vi "System Semaphore Query.vi"(0 "SemaphoreHandle":u16 format="%.0x", 1 "error in (no error)":errorcluster) -> (2 "State String":string, 3 "State":i32, 4 "PreviousCount":i32, 5 "error out":errorcluster)   [LabVIEW 2011]
uses:
  kernel32.dll
panel:
  in  "PreviousCount in":i32
  # "Returns 0, 1, or -1 for Semaphore Unlocked, Locked, or Non-existent"
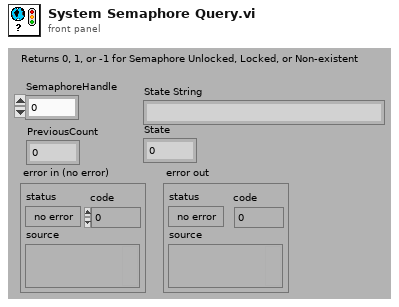
[diagram p1: front panel]
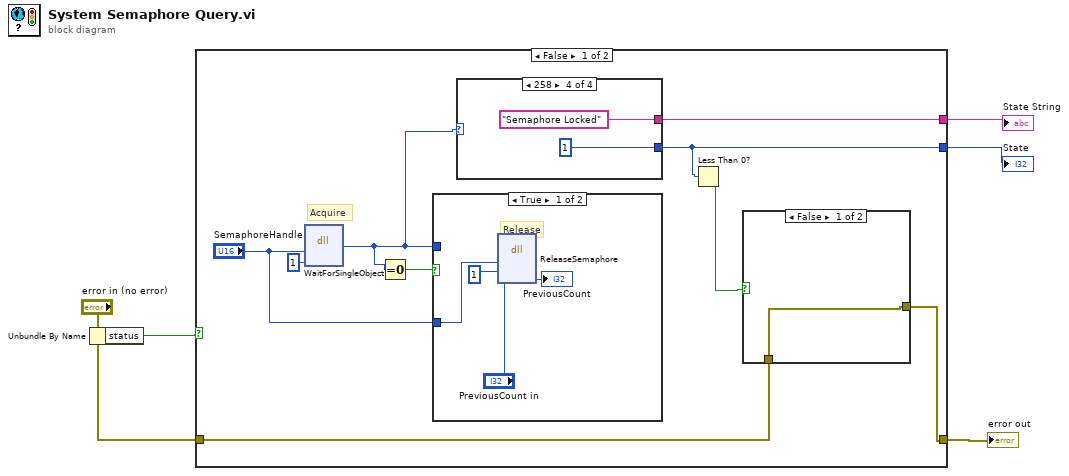
[diagram p0: block diagram]
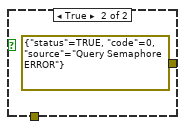
[diagram p3: hidden frame]
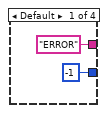
[diagram p4: hidden frame]
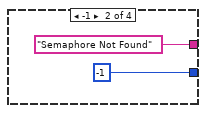
[diagram p5: hidden frame]
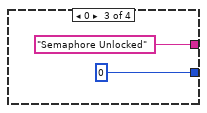
[diagram p6: hidden frame]
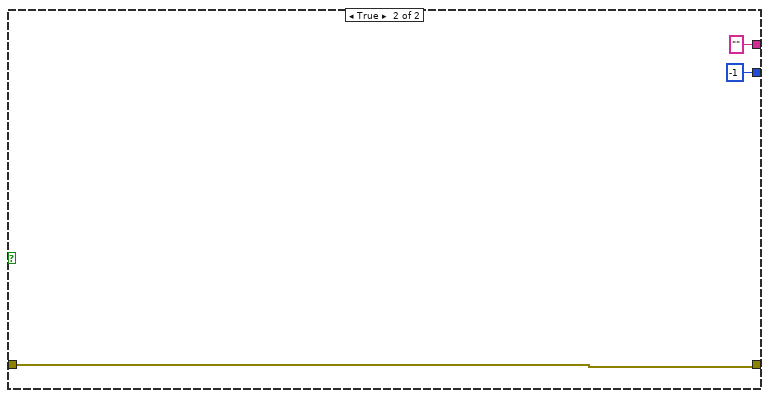
[diagram p7: hidden frame]
diagram:
  n1 = Unbundle By Name("error in (no error)") -> ("status"=w4:bool)
  n2 = case shown="False" w4 {
    tunnel: "error in (no error)" -> [w9 w31]
    tunnel: [w8 w31] -> w1
    tunnel: [w12 ""] -> w3
    tunnel: [w11 -1] -> w2
    frame False {
      # "Acquire"
      n3 = dll-call lib="kernel32.dll" fn="WaitForSingleObject"("SemaphoreHandle"="SemaphoreHandle", "Timeoutms"=u16 1) -> (w7:i16)  [unwired: 5 in, 2 out]
      n4 = Equal To 0?(x=w7) -> (x = 0?=w6:bool)
      n5 = case shown="True" w6 {
        tunnel: "SemaphoreHandle" -> [w18 _]
        tunnel: w7 -> [_ _]
        frame True {
          # "Release"
          n6 = dll-call lib="kernel32.dll" fn="ReleaseSemaphore"("SemaphoreHandle"=w18, "ReleaseCount"=1, "PreviousCount"="PreviousCount in") -> ("PreviousCount"=→"PreviousCount":i32)  [unwired: 6 in, 2 out]
        }
        frame False {
        }
      }
      n7 = case shown="258" w7 {
        tunnel: ["ERROR" "Semaphore Not Found" "Semaphore Unlocked" "Semaphore Locked"] -> w12
        tunnel: [-1 -1 0 1] -> w11
        frame Default {
        }
        frame -1 {
        }
        frame 0 {
        }
        frame 258 {
        }
      }
      n8 = Less Than 0?(x=w11) -> (x < 0?=w10:bool)
      n9 = case shown="False" w10 {
        tunnel: [w19 errorcluster {"status"=TRUE, "code"=0, "source"="Query Semaphore ERROR"} ("error out")] -> w8
        tunnel: w9 -> [w19 _]
        frame False {
        }
        frame True {
        }
      }
    }
    frame True {
    }
  }
  "error out" <- w1
  "State" <- w2
  "State String" <- w3
